vi "AcqTimestampTracepoint.vi"(7 "Qbus":refnum<class "Qbus.lvclass">, 10 "Location":i32, 11 "timestamp log string":string) -> ()   [LabVIEW 2017]
uses:
  <vilib>/addons/TraceLogger/TraceLogger.lvlib
  <vilib>/addons/Qbus/Qbus.lvclass
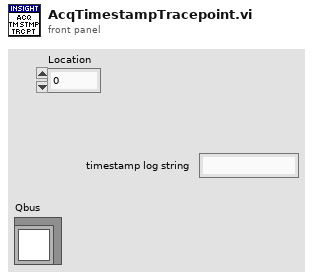
[diagram p1: front panel]
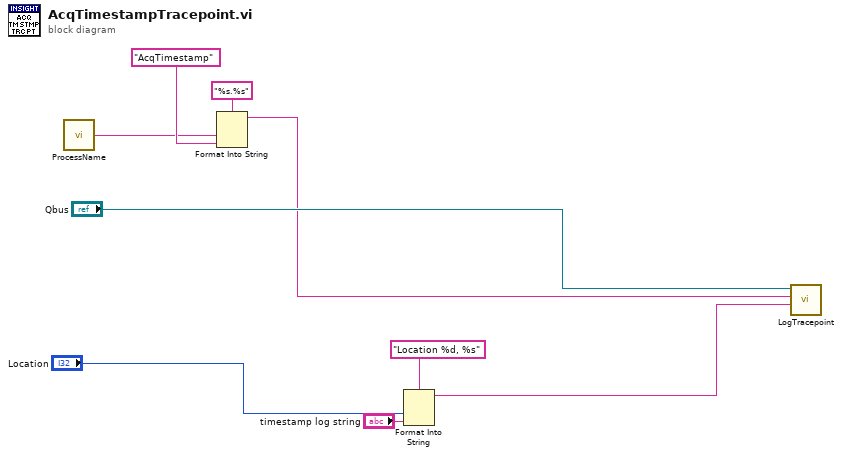
[diagram p0: block diagram]
diagram:
  n1 = call <vilib>:"ProcessName.vi"() -> ("process name"=w2:string)  [unwired: 5 in]
  n2 = Format Into String(format string="%s.%s", w2, "AcqTimestamp" ("tracepoint")) -> (resulting string=w5:string)  [unwired: 2 in, 1 out]
  n3 = Format Into String(format string="Location %d, %s", "Location", "timestamp log string") -> (resulting string=w3:string)  [unwired: 2 in, 1 out]
  n4 = call <vilib>:"LogTracepoint.vi"("log string"=w3, "tracepoint"=w5, "qbus in"="Qbus") -> ()  [unwired: 7 in, 2 out]
